vi "Element Type.vi"(11 "BluelinesRedlines in":refnum<class "BluelinesRedlines.lvclass">) -> (2 "Element Type":string)   [LabVIEW 2020, in "VolatusGUIElements.lvlib" / "BluelinesRedlines.lvclass"]
uses:
  BluelinesRedlines.lvclass
  BluelinesRedlines.lvclass/BluelinesRedlines.ctl
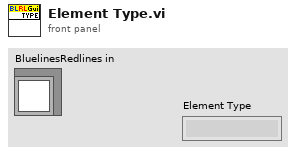
[diagram p1: front panel]
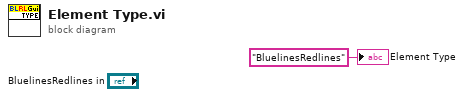
[diagram p0: block diagram]
diagram:
  "Element Type" <- "BluelinesRedlines" ("Element Type")
